vi "Write SP.vi"(8 "error in (no error)":errorcluster, 10 "Enable":bool[](array[boolean]), 11 "Change TEC SPs in":refnum<class "Change TEC Enables.lvclass">) -> (0 "error out":errorcluster, 3 "Change TEC SPs out":refnum<class "Change TEC Enables.lvclass">)   [LabVIEW 2014, in "Change TEC Enables.lvclass"]
uses:
  Change TEC Enables.lvclass
  Change TEC Enables.lvclass/Change TEC Enables.ctl
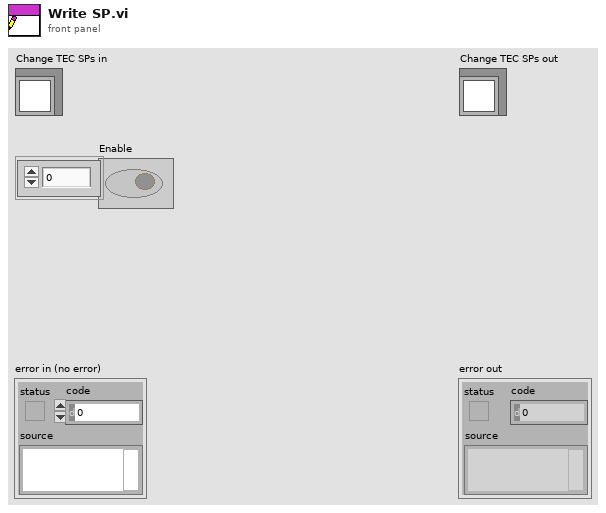
[diagram p1: front panel]
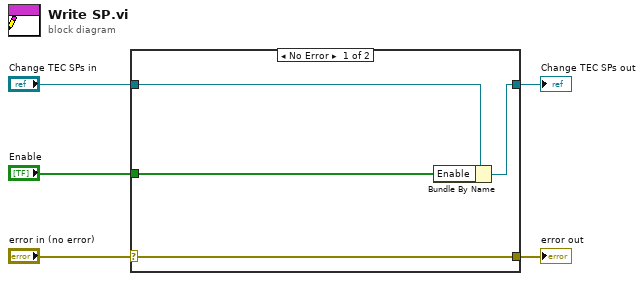
[diagram p0: block diagram]
diagram:
  n1 = case shown="No Error" "error in (no error)" {
    selector: "error in (no error)" -> [w9 w10]
    tunnel: [w9 w10] -> w4
    tunnel: [w7 w11] -> w2
    tunnel: "Change TEC SPs in" -> [w8 w11]
    tunnel: "Enable" -> [w6 _]
    frame No Error {
      n2 = Bundle By Name(cluster=w8, "Enable"=w6) -> (w7:refnum<class "Change TEC Enables.lvclass">)
    }
    frame Error {
    }
  }
  "error out" <- w4
  "Change TEC SPs out" <- w2
